vi "Rename Copyright Year.vi"(8 "error in (no error)":errorcluster, 10 "seconds since 1Jan1904":timestamp, 11 "CSM-Helper in":refnum<class "CSM-Helper.lvclass">) -> (0 "error out":errorcluster, 3 "CSM-Helper out":refnum<class "CSM-Helper.lvclass">)   [LabVIEW 2017, in "CSM-Helper.lvclass"]
uses:
  CSM-Helper.lvclass
  CSM-Helper.lvclass/CSM-Helper.ctl
  Properties/Read While Loop Ref.vi
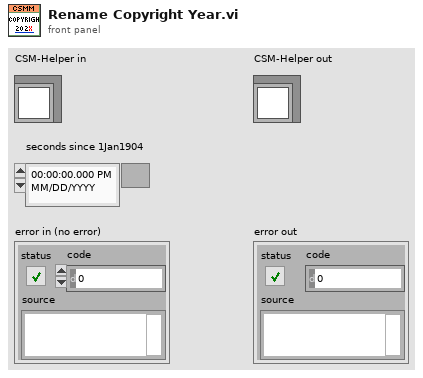
[diagram p1: front panel]
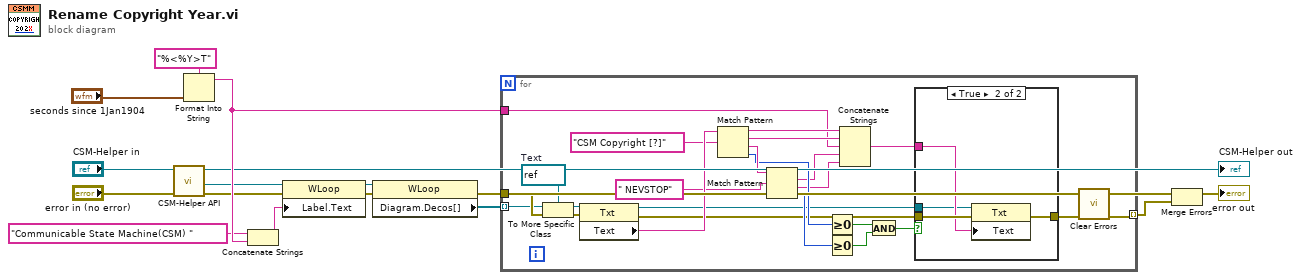
[diagram p0: block diagram]
diagram:
  n1 = call-poly "CSM-Helper API.vi"("error in (no error)"="error in (no error)", "CSM-Helper in"="CSM-Helper in") -> ("error out"=w1:errorcluster, "While Loop"=w2:refnum<vi>, "CSM-Helper out"=→"CSM-Helper out":refnum<class "CSM-Helper.lvclass">)  [unwired: 7 in]
  n2 = Format Into String(format string="%<%Y>T", "seconds since 1Jan1904") -> (resulting string=w16:string)  [unwired: 2 in, 1 out]
  n3 = Concatenate Strings("Communicable State Machine(CSM) " ("string"), w16) -> (w14:string)
  n4 = property class="WLoop"(reference=w2, error in=w1, "Label.Text"=w14) -> (reference out=w9:refnum<vi>, error out=w7:errorcluster)
  n5 = property class="WLoop"(reference=w9, error in=w7) -> (error out=w10:errorcluster, "Diagram.Decos[]"=w11:refnum<vi>[])  [unwired: 1 out]
  n6 = for {
    tunnel: w10 -> [w40]
    tunnel: w11 -> [w39] mode=indexing
    tunnel: [w35] -> w13 mode=indexing
    tunnel: w16 -> [w22]
    w38 = refnum<vi> refnum  # Text
    n7 = To More Specific Class(target class=w38, reference=w39, error in=w40) -> (specific class reference=w37:refnum<vi>, error out=w36:errorcluster)
    n8 = property class="Txt"(reference=w37, error in=w36) -> (reference out=w17:refnum<vi>, error out=w26:errorcluster, "Text"=w34:string)
    n9 = Match Pattern(string=w34, regular expression="CSM Copyright [?]") -> (before substring=w24:string, match substring=w23:string, after substring=w32:string, offset past match=w30:i32)  [unwired: 1 in]
    n10 = Match Pattern(string=w32, regular expression=" NEVSTOP") -> (match substring=w21:string, after substring=w20:string, offset past match=w29:i32)  [unwired: 1 in, 1 out]
    n11 = Greater Or Equal To 0?(x=w30) -> (x >= 0?=w28:bool)
    n12 = Greater Or Equal To 0?(x=w29) -> (x >= 0?=w27:bool)
    n13 = Concatenate Strings(w24, w23, w22, w21, w20) -> (w19:string)
    n14 = And(x=w28, y=w27) -> (x .and. y?=w18:bool)
    n15 = case shown="True" w18 {
      tunnel: w26 -> [w41 w45]
      tunnel: [w41 w44] -> w25
      tunnel: w19 -> [_ w43]
      tunnel: w17 -> [_ w42]
      frame False {
      }
      frame True {
        n16 = property class="Txt"(reference=w42, error in=w45, "Text"=w43) -> (error out=w44:errorcluster)  [unwired: 1 out]
      }
    }
    n17 = call <vilib>:"Clear Errors.vi"("error in (no error)"=w25) -> ("error out"=w35:errorcluster)  [unwired: 5 in, 1 out]
  }
  n18 = Merge Errors(w10, w13) -> (→"error out":errorcluster)
